vi "IntrumentOpener.vi"(0 "Input Array":dbl[](array[numeric])) -> (1 "Instrument Data":T2, 2 "Lowest RMS b":T1, 3 "RMS Values":T3 {"RMS Harmonica" format="%0.2f"; "RMS Mandolin" format="%0.2f"; "RMS Guitar" format="%0.2f"; "RMS Tone Generator" format="%0.2f"})   [LabVIEW 2015]
uses:
  <vilib>/Analysis/5stat.llb/RMS (DBL).vi
  <vilib>/Utility/file.llb/Read Delimited Spreadsheet (DBL).vi
  <vilib>/Analysis/NI_AALPro.lvlib
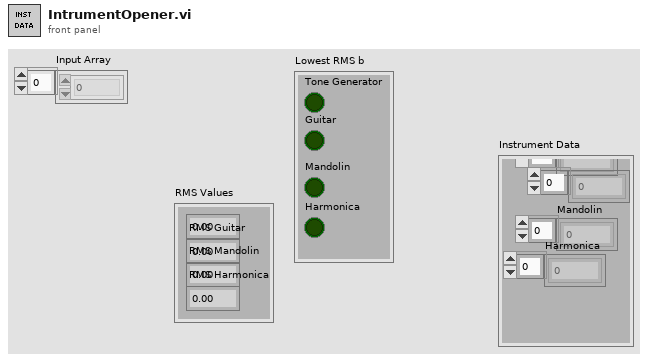
[diagram p1: front panel]
types:
  T1 = cluster{"Tone Generator":bool, "Guitar":bool, "Mandolin":bool, "Harmonica":bool}
  T2 = cluster{"\nTone Generator":dbl[], "Guitar":dbl[], "Mandolin":dbl[], "Harmonica":dbl[]}
  T3 = cluster{"RMS Tone Generator":dbl, "RMS Guitar":dbl, "RMS Mandolin":dbl, "RMS Harmonica":dbl}
  T4 = cluster{"x/y":dbl[], "x/y":dbl[], "x/y":dbl[], "x/y":dbl[]}
  T5 = cluster{"rms value":dbl, "rms value":dbl, "rms value":dbl, "rms value":dbl}
  T6 = cluster{"[0]":bool, "[1]":bool, "[2]":bool, "[3]":bool}
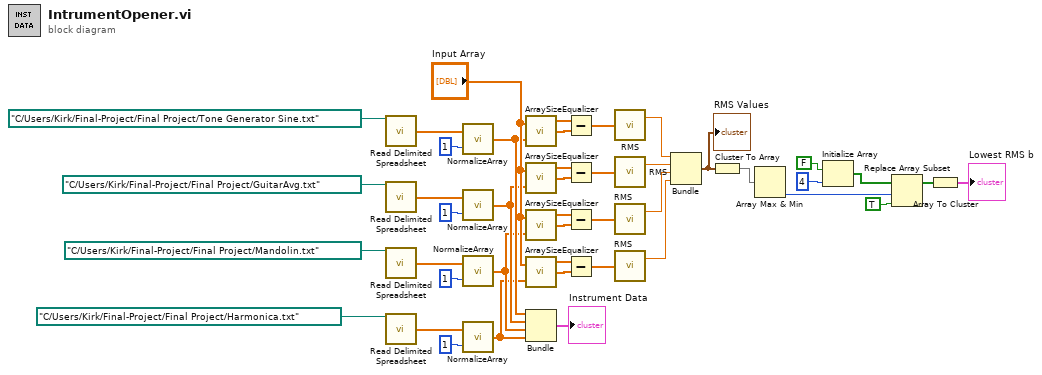
[diagram p0: block diagram]
diagram:
  n1 = call-poly <vilib>:"Read Delimited Spreadsheet.vi"("file path (dialog if empty)"=path "C:/Users/Kirk/Final-Project/Final Project/Tone Generator Sine.txt" ("Path")) -> ("first row"=w35:dbl[])  [unwired: 9 in, 5 out]
  n2 = call-poly <vilib>:"Read Delimited Spreadsheet.vi"("file path (dialog if empty)"=path "C:/Users/Kirk/Final-Project/Final Project/GuitarAvg.txt" ("Path")) -> ("first row"=w34:dbl[])  [unwired: 9 in, 5 out]
  n3 = call-poly <vilib>:"Read Delimited Spreadsheet.vi"("file path (dialog if empty)"=path "C:/Users/Kirk/Final-Project/Final Project/Mandolin.txt" ("Path")) -> ("first row"=w36:dbl[])  [unwired: 9 in, 5 out]
  n4 = call-poly <vilib>:"Read Delimited Spreadsheet.vi"("file path (dialog if empty)"=path "C:/Users/Kirk/Final-Project/Final Project/Harmonica.txt" ("Path")) -> ("first row"=w37:dbl[])  [unwired: 9 in, 5 out]
  n5 = call "NormalizeArray.vi"("index"=1, "Array"=w35) -> ("x/y"=w16:dbl[])
  n6 = call "NormalizeArray.vi"("index"=1, "Array"=w34) -> ("x/y"=w15:dbl[])
  n7 = call "NormalizeArray.vi"("index"=1, "Array"=w36) -> ("x/y"=w14:dbl[])
  n8 = call "NormalizeArray.vi"("index"=1, "Array"=w37) -> ("x/y"=w13:dbl[])
  n9 = call "ArraySizeEqualizer.vi"("Array1in"="Input Array", "Array 2in"=w16) -> ("Array1out"=w30:dbl[], "Array2out"=w29:dbl[])  [unwired: 1 out]
  n10 = call "ArraySizeEqualizer.vi"("Array1in"="Input Array", "Array 2in"=w15) -> ("Array1out"=w33:dbl[], "Array2out"=w32:dbl[])  [unwired: 1 out]
  n11 = call "ArraySizeEqualizer.vi"("Array1in"="Input Array", "Array 2in"=w14) -> ("Array1out"=w27:dbl[], "Array2out"=w26:dbl[])  [unwired: 1 out]
  n12 = call "ArraySizeEqualizer.vi"("Array1in"="Input Array", "Array 2in"=w13) -> ("Array1out"=w24:dbl[], "Array2out"=w23:dbl[])  [unwired: 1 out]
  n13 = Bundle("x/y"=w16, "x/y"=w15, "x/y"=w14, "x/y"=w13) -> (→"Instrument Data":T4)  [unwired: 1 in]
  n14 = Subtract(x=w30, y=w29) -> (x-y=w28:dbl[])
  n15 = Subtract(x=w33, y=w32) -> (x-y=w31:dbl[])
  n16 = Subtract(x=w27, y=w26) -> (x-y=w25:dbl[])
  n17 = Subtract(x=w24, y=w23) -> (x-y=w22:dbl[])
  n18 = call-poly <vilib>:"RMS.vi"("X"=w28) -> ("rms value"=w20:dbl)  [unwired: 1 out]
  n19 = call-poly <vilib>:"RMS.vi"("X"=w31) -> ("rms value"=w19:dbl)  [unwired: 1 out]
  n20 = call-poly <vilib>:"RMS.vi"("X"=w25) -> ("rms value"=w18:dbl)  [unwired: 1 out]
  n21 = call-poly <vilib>:"RMS.vi"("X"=w22) -> ("rms value"=w17:dbl)  [unwired: 1 out]
  n22 = Bundle("rms value"=w20, "rms value"=w19, "rms value"=w18, "rms value"=w17) -> (w7:T5)  [unwired: 1 in]
  "RMS Values" <- w7
  n23 = Cluster To Array(cluster=w7) -> (array=w6:dbl[])
  n24 = Array Max & Min(array=w6) -> (min index (indices)=w5:i32)  [unwired: 3 out]
  n25 = Initialize Array(FALSE, 4 ("dimension size")) -> (w3:bool[])
  n26 = Replace Array Subset(array=w3, new element=TRUE, index=w5) -> (w2:bool[])
  n27 = Array To Cluster(array=w2) -> (cluster=→"Lowest RMS b":T6)
